vi "Get Selected Type.vi"(0 "Select Type":T1, 11 "error in (no error)":errorcluster) -> (4 "Selected Type Pattern":string, 15 "error out":errorcluster)   [LabVIEW 2014, in "SLL Add Copyright.lvlib"]
uses:
  SLL Add Copyright.lvlib
  Typedefs/Select Type.ctl
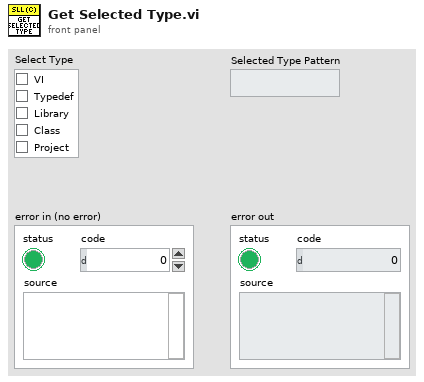
[diagram p1: front panel]
types:
  T1 = typedef "SLL Add Copyright.lvlib/Select Type.ctl" = cluster{"vi":bool, "ctl":bool, "lvlib":bool, "lvclass":bool, "lvproj":bool}
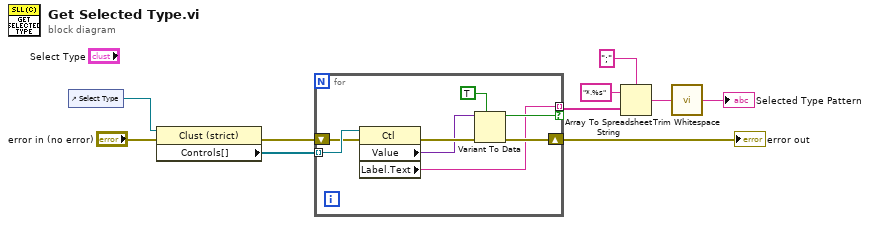
[diagram p0: block diagram]
diagram:
  n1 = control-ref of="Select Type"() -> (w6:refnum<vi>)
  n2 = property class="Clust (strict)"(reference=w6, error in="error in (no error)") -> (error out=w9:errorcluster, "Controls[]"=w10:refnum<vi>[])  [unwired: 1 out]
  n3 = for {
    tunnel: w10 -> [w18] mode=indexing
    tunnel: [w11] -> w5 mode=indexing if=w15
    shift-right: [w13] -> w7
    shift-left: w9 -> [w14]
    n4 = property class="Ctl"(reference=w18, error in=w14) -> (error out=w17:errorcluster, "Value"=w12:variant, "Label.Text"=w11:string)  [unwired: 1 out]
    n5 = Variant To Data(error in=w17, type=TRUE, Variant=w12) -> (data=w15:bool, error out=w13:errorcluster)
  }
  "error out" <- w7
  n6 = Array To Spreadsheet String(delimiter (Tab)=";", array=w5, 3:"*.%s" ("format string")) -> (spreadsheet string=w2:string)
  n7 = call <vilib>:"Trim Whitespace.vi"("string"=w2) -> ("trimmed string"=→"Selected Type Pattern":string)  [unwired: 1 in]
